vi "initializeORCA.vi"() -> (2 "Handle out":u32, 3 "x != 0?":bool)   [LabVIEW 2016]
uses:
  <vilib>/Utility/error.llb/DialogType.ctl
panel:
  in  "Value":dbl(slide) min=1.0 max=14.0 scale=1.0..14.0
  in  "Text Value":dbl(ring) items=["AREA"=1.0, "SPLIT VIEW"=14.0]
  in  "Parameter":u32(ring)=4212128 items=["SENSOR MODE"=4212128, "READOUT SPEED"=4211872, "READOUT DIRECTION"=4211904, "COLORTYPE"=4342960, "BIT PER CHANNEL"=4342976, "TRIGGER SOURCE"=1066144, "TRIGGER MODE"=1066400, "TRIGGER ACTIVE"=1066160, "TRIGGER GLOBAL EXPOSURE"=2049680, "TRIGGER POLARITY"=1066416, "TRIGGER TIMES"=1066448, "TRIGGER DELAY"=1066480, "INTERNAL TRIGGER HANDLING"=1066496, "EXPOSURE TIME CONTROL"=2049216, "EXPOSURE TIME"=2049184, "DEFECT CORRECT MODE"=4670368, "BINNING"=4215968, "SUBARRAY HPOS"=4220064, "SUBARRAY HSIZE"=4220080, "SUBARRAY VPOS"=4220096, "SUBARRAY VSIZE"=4220112, "SUBARRAY MODE"=4220128, "TIMING READOUT TIME"=4223904, "TIMING CYCLIC TRIGGER PERIOD"=4223920, "TIMING MIN TRIGGER BLANKING"=4223936, "TIMING MIN TRIGGER INTERVAL"=4223968, "TIMING GLOBAL EXPOSURE DELAY"=4224032, "TIMING EXPOSURE"=4223984, "TIMING INVALID EXPOSURE PERIOD"=4224000, "INTERNAL FRAME RATE"=4225952, "INTERNAL FRAME INTERVAL"=4225968, "FRAMEBUNDLE MODE"=4346784, "FRAMEBUNDLE NUMBER"=4346800, "FRAMEBUNDLE ROWBYTES"=4346816, "FRAMEBUNDLE FRAME STEP BYTES"=4346832, "IMAGE WIDTH"=4343200, "IMAGE HEIGHT"=4343216, "IMAGE ROWBYTES"=4343232, "IMAGE FRAMEBYTES"=4343248, "IMAGE TOP OFFSET BYTES"=4343264, "IMAGE PIXEL TYPE"=4343296, "IMAGE CAMERA STAMP"=4343440, "BUFFER ROWBYTES"=4343488, "BUFFER FRAMEBYTES"=4343504, "BUFFER TOP OFFSET BYTES"=4343520, "BUFFER PIXEL TYPE"=4343536, "RECORD FIXED BYTES PER FILE"=4343712, "RECORD FIXED BYTES PER SESSION"=4343728, "RECORD FIXED BYTES PER FRAME"=4343744, "NUMBER OF OUTPUT TRIGGER CONNECTOR"=1852320, "OUTPUT TRIGGER CHANNEL SYNC"=1852352, "OUTPUT TRIGGER PROGRAMABLE START"=1852384, "OUTPUT TRIGGER SOURCE[0]"=1852576, "OUTPUT TRIGGER POLARITY[0]"=1852592, "OUTPUT TRIGGER ACTIVE[0]"=1852608, "OUTPUT TRIGGER DELAY[0]"=1852624, "OUTPUT TRIGGER PERIOD[0]"=1852640, "OUTPUT TRIGGER KIND[0]"=1852656, "SYSTEM ALIVE"=16728992, "CONVERSION FACTOR COEFF"=16786336, "CONVERSION FACTOR OFFSET"=16786352, "NUMBER OF VIEW"=4343120, "IMAGE DETECTOR PIXEL WIDTH"=4344736, "IMAGE DETECTOR PIXEL HEIGHT"=4344752, "TIME STAMP PRODUCER"=4279712, "FRAME STAMP PRODUCER"=4279728]
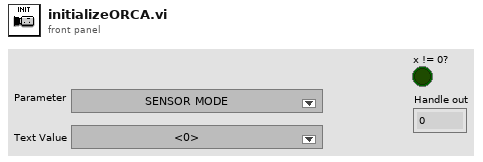
[diagram p1: front panel]
types:
  T1 = typedef "DialogType.ctl" = u16
  T2 = enum8{"Enabled", "Disabled", "Disabled and Grayed Out"}
  T3 = cluster{"Function Name":string, "Function ID":dbl}[]
  T4 = cluster{"Function Name":string, "Function ID":dbl}
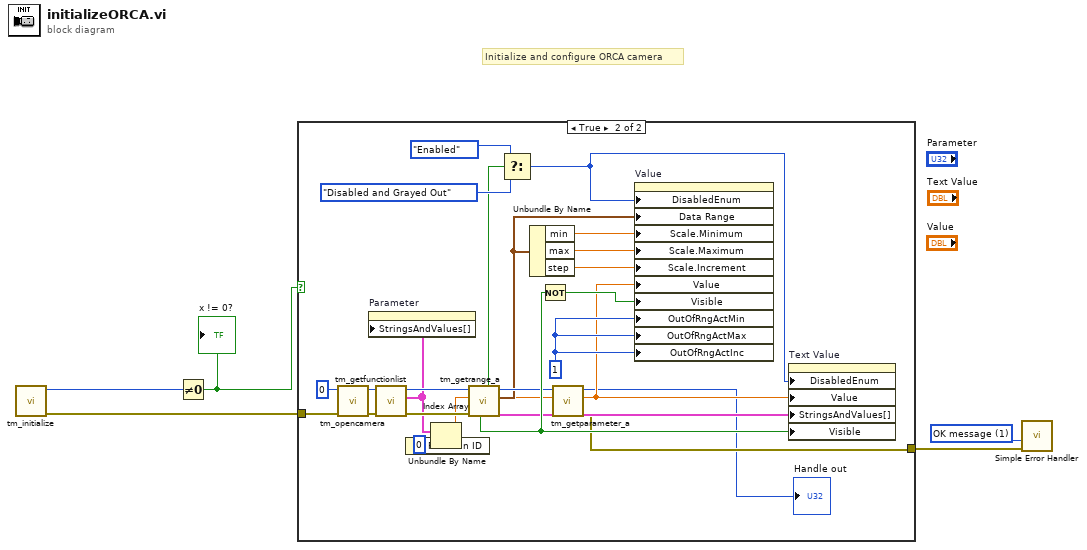
[diagram p0: block diagram]
diagram:
  w3 = T1 1 items=["no dialog", "OK message", "continue or stop message", "OK message + warnings", "continue/stop + warnings"] ("type of dialog (OK msg:1)")
  # "Initialize and configure ORCA camera"
  n1 = call <userlib>:"tm_initialize.vi"() -> ("error out"=w1:errorcluster, "Number Of Cameras"=w5:u32)  [unwired: 8 in, 2 out]
  n2 = Not Equal To 0?(x=w5) -> (x != 0?=w2:bool)
  "x != 0?" <- w2
  n3 = case shown="True" w2 {
    tunnel: w1 -> [w6 w8]
    tunnel: [w6 w9] -> w4
    frame False {
    }
    frame True {
      w23 = u8 1 ("Out Of Range Action:Increment")
      n4 = call <userlib>:"tm_opencamera.vi"("error in (no error)"=w8, "Camera Index"=u32 0) -> ("error out"=w32:errorcluster, "Handle out"=w33:u32)  [unwired: 7 in, 1 out]
      n5 = call <userlib>:"tm_getfunctionlist.vi"("error in (no error)"=w32, "Handle in"=w33) -> ("error out"=w20:errorcluster, "Function List"=w10:T3, "Handle out"=w21:u32)  [unwired: 7 in]
      n6 = property on="Parameter" class="Ring (strict)"("StringsAndValues[]"=w10) -> ()  [unwired: 2 in, 2 out]
      n7 = Index Array(array=w10, index=0) -> (element=w12:T4)
      n8 = Unbundle By Name(w12) -> ("Function ID"=w11:dbl)
      n9 = call <userlib>:"tm_getrange_a.vi"("error in (no error)"=w20, "Parameter"=w11, "Handle in"=w21) -> ("error out"=w14:errorcluster, "Range"=w15:cluster{"min":dbl, "max":dbl, "step":dbl}, "Handle out"=w16:u32, "Value Names"=w18:cluster{"Name":string, "Value":dbl}[], "Writable"=w17:bool, "Text Values"=w19:bool)  [unwired: 2 in, 1 out]
      n10 = Select(t=T2."Enabled" ("Disabled"), s=w17, f=T2."Disabled and Grayed Out" ("Disabled")) -> (s? t:f=w28:T2)
      n11 = Unbundle By Name(w15) -> ("min"=w27:dbl, "max"=w26:dbl, "step"=w25:dbl)
      n12 = Not(x=w19) -> (.not. x?=w24:bool)
      n13 = call <userlib>:"tm_getparameter_a.vi"("error in (no error)"=w14, "Parameter"=w11, "Handle in"=w16) -> ("error out"=w9:errorcluster, "Value out"=w22:dbl, "Handle out"=→"Handle out":u32)  [unwired: 6 in]
      n14 = property on="Value" class="Slide (strict)"("DisabledEnum"=w28, "Data Range"=w15, "Scale.Minimum"=w27, "Scale.Maximum"=w26, "Scale.Increment"=w25, "Value"=w22, "Visible"=w24, "OutOfRngActMin"=w23, "OutOfRngActMax"=w23, "OutOfRngActInc"=w23) -> ()  [unwired: 2 in, 2 out]
      n15 = property on="Text Value" class="Ring (strict)"("DisabledEnum"=w28, "Value"=w22, "StringsAndValues[]"=w18, "Visible"=w19) -> ()  [unwired: 2 in, 2 out]
    }
  }
  n16 = call <vilib>:"Simple Error Handler.vi"("type of dialog (OK msg:1)"=w3, "error in (no error)"=w4) -> ()  [unwired: 3 in, 5 out]
